vi "SwTmr Settings Dialog.vi"(8 "error in (no error)":errorcluster, 11 "Configuration in":T1={"Hardware Configuration"={"Physical Channel"="", "Maximum Input"=0.0, "Minimum Input"=0.0, "Sample Rate"=0.0, "Number of Samples"=0}, "Analysis Configuration"={"Statistics"=TRUE}, "New Data Behavior"=enum."Replace", "Time-Voltage transfer function file path (dialog if empty)"=path "", "Cell (V) Error Upper"=0.0, "Cell (V) Error Lower (type \"-\")"=0.0}) -> (0 "error out":errorcluster, 2 "UI Refresh Needed?":bool, 3 "Configuration out":T1={"Hardware Configuration"={"Physical Channel"="", "Maximum Input"=0.0, "Minimum Input"=0.0, "Sample Rate"=0.0, "Number of Samples"=0}, "Analysis Configuration"={"Statistics"=TRUE}, "New Data Behavior"=enum."Replace", "Time-Voltage transfer function file path (dialog if empty)"=path "", "Cell (V) Error Upper"=0.0, "Cell (V) Error Lower (type \"-\")"=0.0})   [LabVIEW 2017]
doc: "Dialog for selecting user specified settings."
uses:
  controls/SwTmr User Specified Data.ctl
  controls/SwTmr HW Configuration.ctl
  controls/SwTmr Analysis Configuration.ctl
  controls/SwTmr New Data Behavior.ctl
  controls/SwTmr Transfer Func File Path.ctl
panel:
  in  "Cell (V) Error Lower (type \"-\")":dbl
  in  "Cell (V) Error Upper":dbl
  in  "Time-Voltage transfer function file path":path
  in  "Number of Samples/Ch":i32=1000
  in  "Sample Rate":dbl=10000.0
  in  "Minimum Input":dbl=-10.0
  in  "Maximum Input":dbl=10.0
  in  "Physical Channel":tag="Dev1/ai0"
  in  "New Data Behavior":u16(ring) items=["Replace", "Overlay", "Append"]
  in  "Cancel Button":bool
  in  "OK Button":bool
  # "Tab delimited Text File:Time in 1st col, Voltage \nin 2nd column  ascending"
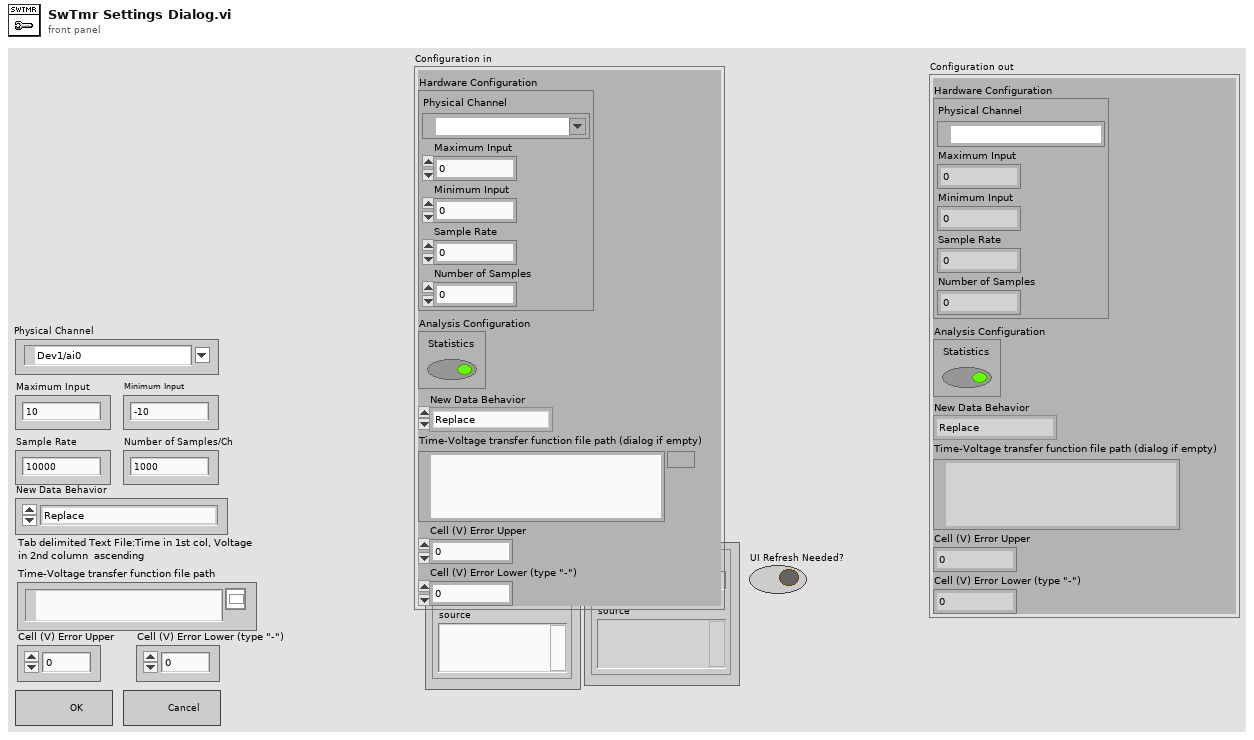
[diagram p1: front panel]
types:
  T1 = typedef "SwTmr User Specified Data.ctl" = cluster{"Hardware Configuration":T2, "Analysis Configuration":T3, "New Data Behavior":T4, "Time-Voltage transfer function file path (dialog if empty)":T5, "Cell (V) Error Upper":dbl, "Cell (V) Error Lower (type \"-\")":dbl}
  T2 = typedef "SwTmr HW Configuration.ctl" = cluster{"Physical Channel":tag, "Maximum Input":dbl, "Minimum Input":dbl, "Sample Rate":dbl, "Number of Samples":i32}
  T3 = typedef "SwTmr Analysis Configuration.ctl" = cluster{"Statistics":bool}
  T4 = typedef "SwTmr New Data Behavior.ctl" = enum16{"Replace", "Overlay", "Append"}
  T5 = typedef "SwTmr Transfer Func File Path.ctl" = path
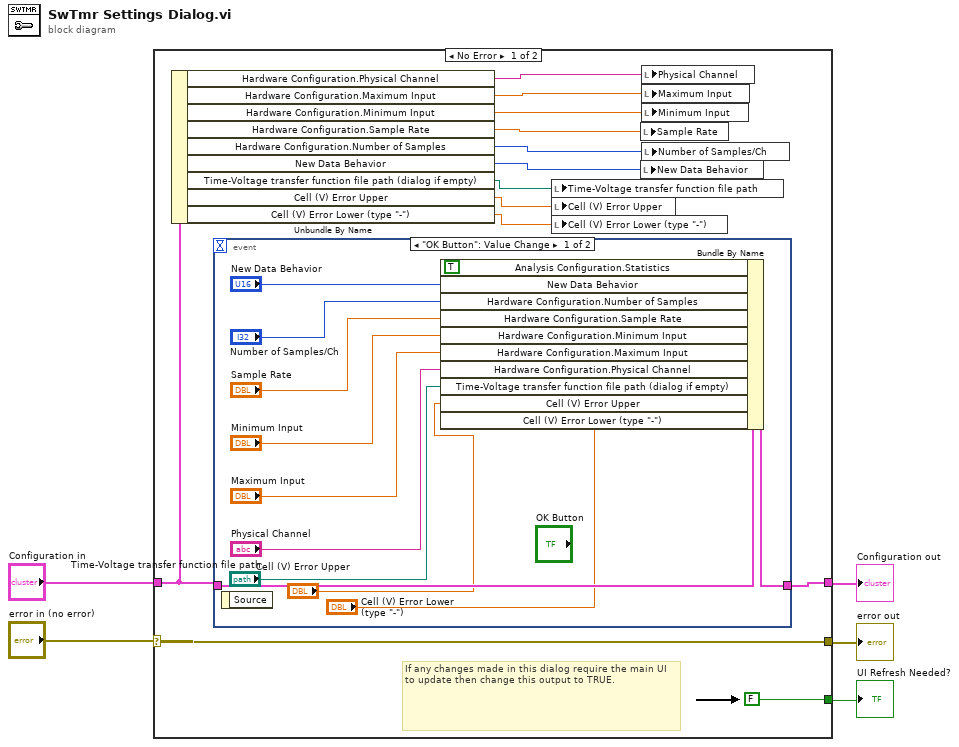
[diagram p0: block diagram]
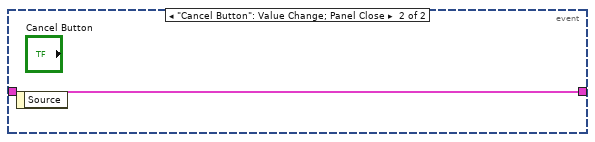
[diagram p2: hidden frame]
diagram:
  n1 = case shown="No Error" "error in (no error)" {
    selector: "error in (no error)" -> [w16 w33]
    tunnel: [w16 w33] -> w4
    tunnel: "Configuration in" -> [w15 w32]
    tunnel: [w18 w32] -> w2
    tunnel: [FALSE ("UI Refresh Needed?") _] -> w1
    frame No Error {
      # "If any changes made in this dialog require the main UI to update then change this output to TRUE."
      n2 = Unbundle By Name(w15) -> ("Hardware Configuration.Physical Channel"=w14:tag, "Hardware Configuration.Maximum Input"=w13:dbl, "Hardware Configuration.Minimum Input"=w12:dbl, "Hardware Configuration.Sample Rate"=w11:dbl, "Hardware Configuration.Number of Samples"=w10:i32, "New Data Behavior"=w9:T4, "Time-Voltage transfer function file path (dialog if empty)"=w8:T5, "Cell (V) Error Upper"=w7:dbl, "Cell (V) Error Lower (type \"-\")"=w6:dbl)
      n3 = event shown="[0] \"OK Button\": Value Change" {
        selector: _ -> [_ _]
        dyn-events: _ -> [_ _]
        timeout: _ -> [_ _]
        tunnel: [w30 w31] -> w18
        tunnel: w15 -> [w28 w31]
        event "OK Button": Value Change {
          n4 = event-data() -> ()  [unwired: 1 in, 1 out]
          n5 = Bundle By Name(cluster=w28, "Analysis Configuration.Statistics"=TRUE, "New Data Behavior"="New Data Behavior", "Hardware Configuration.Number of Samples"="Number of Samples/Ch", "Hardware Configuration.Sample Rate"="Sample Rate", "Hardware Configuration.Minimum Input"="Minimum Input", "Hardware Configuration.Maximum Input"="Maximum Input", "Hardware Configuration.Physical Channel"="Physical Channel", "Time-Voltage transfer function file path (dialog if empty)"="Time-Voltage transfer function file path", "Cell (V) Error Upper"="Cell (V) Error Upper", "Cell (V) Error Lower (type \"-\")"="Cell (V) Error Lower (type \"-\")") -> (w30:T1)
        }
        event "Cancel Button": Value Change; Panel Close {
          n6 = event-data() -> ()  [unwired: 1 in, 1 out]
        }
      }
      n7 = local write "Time-Voltage transfer function file path"(w8) -> ()
      n8 = local write "Cell (V) Error Upper"(w7) -> ()
      n9 = local write "Cell (V) Error Lower (type \"-\")"(w6) -> ()
      n10 = local write "Sample Rate"(w11) -> ()
      n11 = local write "New Data Behavior"(w9) -> ()
      n12 = local write "Physical Channel"(w14) -> ()
      n13 = local write "Maximum Input"(w13) -> ()
      n14 = local write "Minimum Input"(w12) -> ()
      n15 = local write "Number of Samples/Ch"(w10) -> ()
    }
    frame Error {
    }
  }
  "UI Refresh Needed?" <- w1
  "error out" <- w4
  "Configuration out" <- w2
